vi "GVMethodenwechsel.vi"() -> ()   [LabVIEW 2010]
panel:
  out "Methodenwechsel?":bool
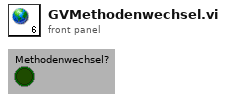
[diagram p1: front panel]
diagram:
